vi "Wireless_Serial_Test.vi"() -> ()   [LabVIEW 2010]
uses:
  <vilib>/Instr/_visa.llb/VISA Configure Serial Port (Instr).vi
panel:
  out "Waveform Chart 13":u32(graph)
  out "Waveform Chart 12":u32(graph)
  out "Waveform Chart 11":u32(graph)
  out "Waveform Chart 10":u32(graph)
  out "Waveform Chart 9":u32(graph)
  out "Check Sum":u32(graph)
  out "Waveform Chart 7":u32(graph)
  out "Waveform Chart 6":u32(graph)
  out "Waveform Chart 5":u32(graph)
  out "Waveform Chart 4":u32(graph)
  out "Waveform Chart 3":u32(graph)
  out "Waveform Chart 2":u32(graph)
  out "Waveform Chart":u32(graph)
  in  "byte count":u32=18
  in  "VISA resource name":refnum<visa-resource-name>="COM4"
  in  "stop":bool
  out "Looped Incoming String":string
  out "Active Channels":string
  out "Source Address":string
  out "Byte Length":dbl
  out "RSSI":dbl
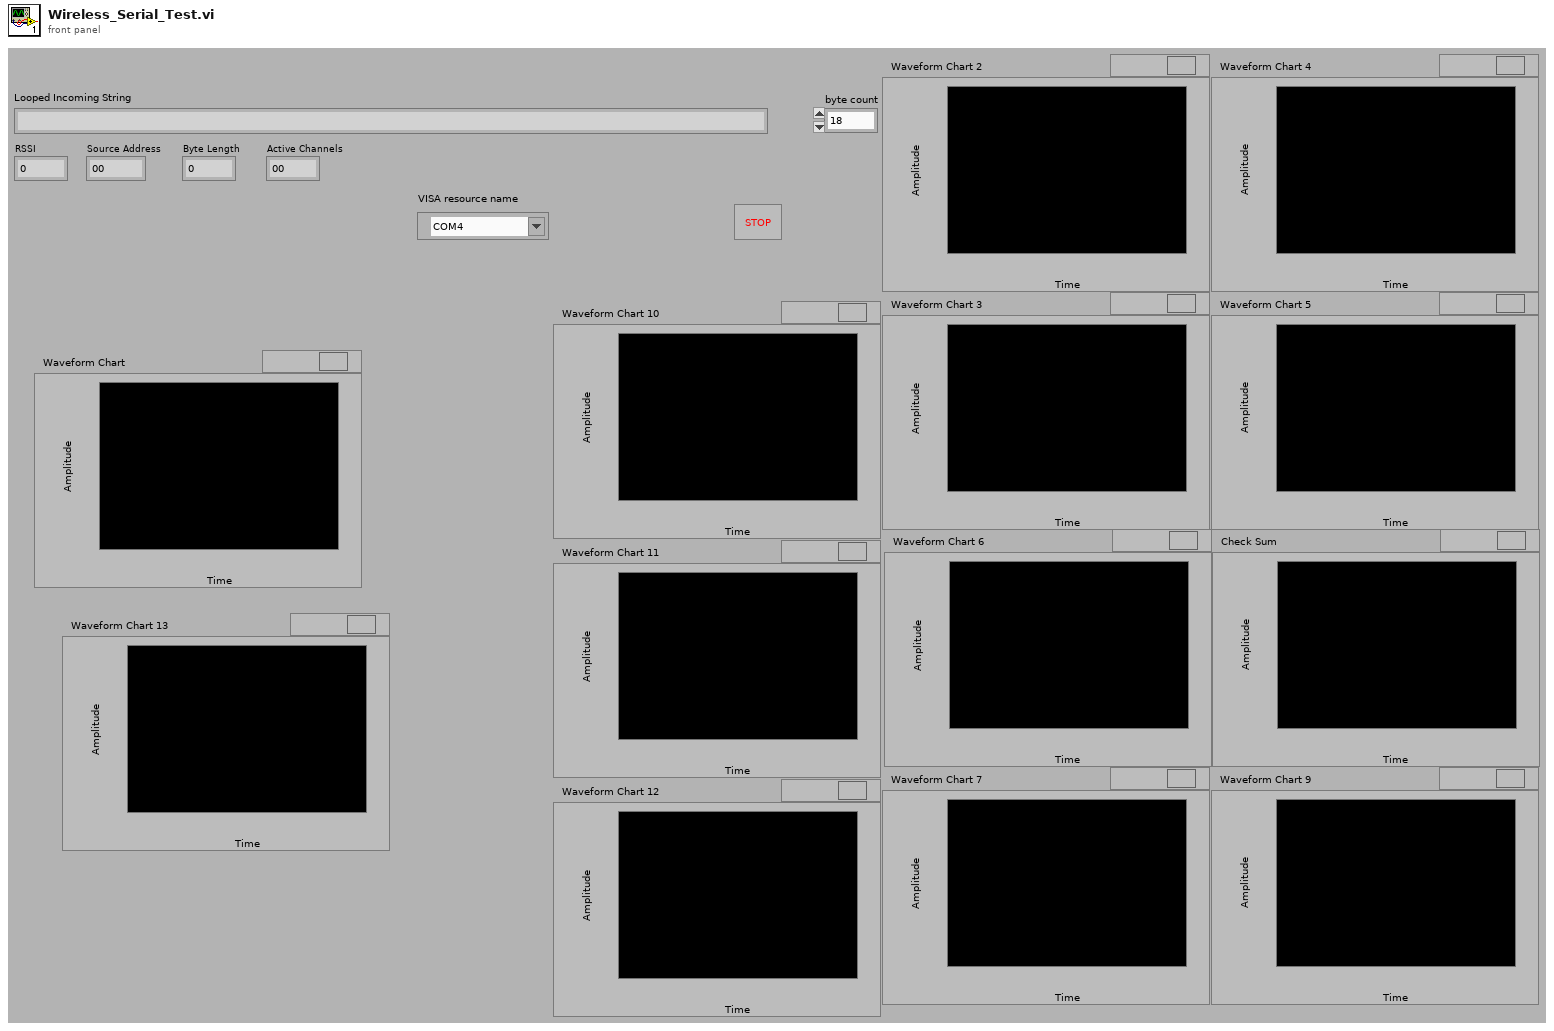
[diagram p1: front panel]
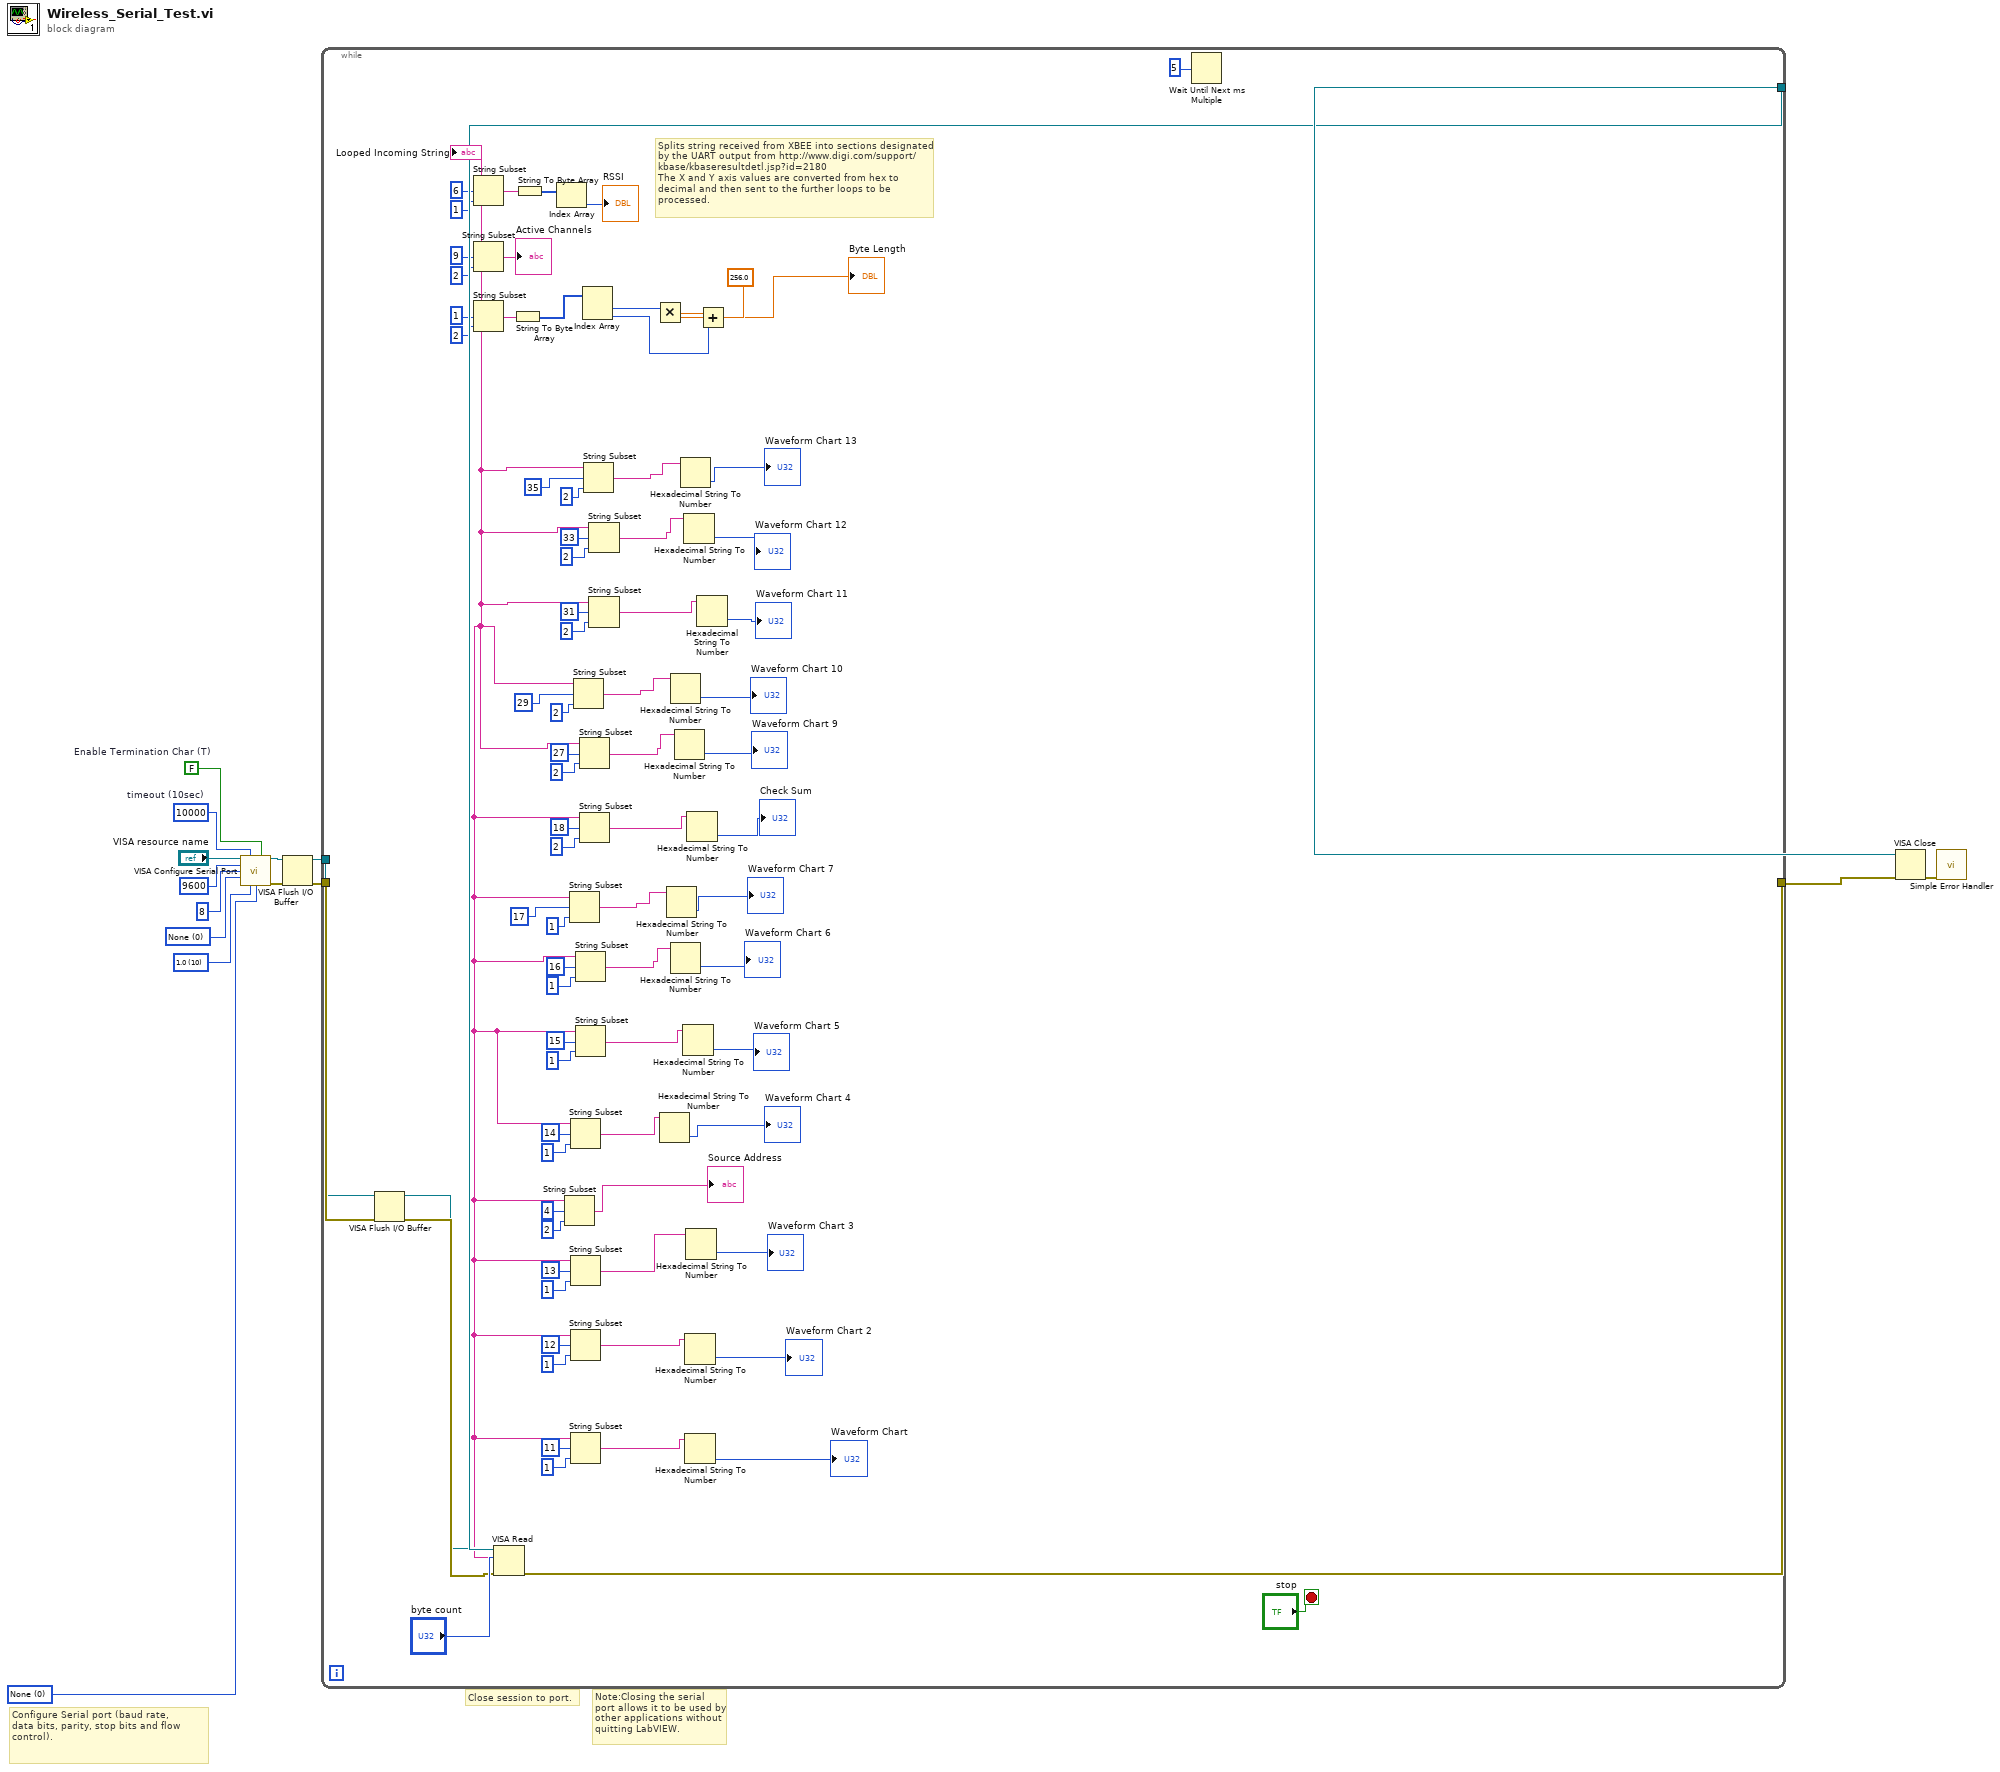
[diagram p0: block diagram]
diagram:
  w4 = u16 0 items=["None"=0, "XON/XOFF"=1, "RTS/CTS"=2, "DTR/DSR"=4] ("flow control")
  w5 = u16 10 items=["1.0"=10, "1.5"=15, "2.0"=20] ("stop bits")
  w8 = u16 0 items=["None", "Odd", "Even", "Mark", "Space"] ("parity")
  w6 = FALSE  # Enable Termination Char (T)
  w7 = u32 10000  # timeout (10sec)
  # "Configure Serial port (baud rate,\ndata bits, parity, stop bits and flow control)."
  # "Note:Closing the serial port allows it to be used by other applications without\nquitting LabVIEW."
  # "Close session to port."
  n1 = call-poly "VISA Configure Serial Port"("VISA resource name"="VISA resource name", "timeout (10sec)"=w7, "Enable Termination\nChar (T)"=w6, "baud rate (9600)"=u32 9600 ("baud rate"), "data bits (8)"=u16 8 ("data bits"), "parity (0:none)"=w8, "stop bits (10: 1 bit)"=w5, "flow control (0:none)"=w4) -> ("VISA resource name out"=w9:refnum<visa-resource-name>, "error out"=w10:errorcluster)  [unwired: 1 in, 5 out]
  n2 = VISA Flush I/O Buffer(VISA resource name=w9, error in (no error)=w10) -> (VISA resource name out=w2:refnum<visa-resource-name>, error out=w1:errorcluster)  [unwired: 1 out]
  n3 = while {
    tunnel: [w97] -> w15
    tunnel: [w96] -> w14
    tunnel: w2 -> [w63]
    tunnel: w1 -> [w64]
    stop <- "stop" stop-if-true
    # "Splits string received from XBEE into sections designated by the UART output from http://www.digi.com/support/kbase/kbaseresultdetl.jsp?id=2180 \nThe X and Y axis values are converted from hex to decimal and then sent to the further loops to be processed."
    n4 = VISA Flush I/O Buffer(VISA resource name=w63, error in (no error)=w64) -> (VISA resource name out=w65:refnum<visa-resource-name>, error out=w66:errorcluster)  [unwired: 1 out]
    n5 = VISA Read(VISA resource name=w65, byte count="byte count", error in (no error)=w66) -> (VISA resource name out=w96:refnum<visa-resource-name>, read buffer=w29:string, error out=w97:errorcluster)  [unwired: 1 out]
    "Looped Incoming String" <- w29
    n6 = String Subset(string=w29, offset (0)=6, length (rest)=1 ("length (rest)")) -> (substring=w68:string)
    n7 = String Subset(string=w29, offset (0)=9, length (rest)=2 ("length (rest)")) -> (substring=→"Active Channels":string)
    n8 = String Subset(string=w29, offset (0)=1, length (rest)=2 ("length (rest)")) -> (substring=w70:string)
    n9 = String To Byte Array(string=w70) -> (unsigned byte array=w72:u8[])
    n10 = String To Byte Array(string=w68) -> (unsigned byte array=w69:u8[])
    n11 = Index Array(array=w69) -> (element=→"RSSI":u8)  [unwired: 1 in]
    n12 = String Subset(string=w29, offset (0)=4, length (rest)=2 ("length (rest)")) -> (substring=→"Source Address":string)
    n13 = String Subset(string=w29, offset (0)=17, length (rest)=1 ("length (rest)")) -> (substring=w54:string)
    n14 = String Subset(string=w29, offset (0)=14, length (rest)=1 ("length (rest)")) -> (substring=w51:string)
    n15 = String Subset(string=w29, offset (0)=13, length (rest)=1 ("length (rest)")) -> (substring=w50:string)
    n16 = String Subset(string=w29, offset (0)=12, length (rest)=1 ("length (rest)")) -> (substring=w49:string)
    n17 = String Subset(string=w29, offset (0)=11, length (rest)=1 ("length (rest)")) -> (substring=w48:string)
    n18 = String Subset(string=w29, offset (0)=29, length (rest)=2 ("length (rest)")) -> (substring=w41:string)
    n19 = String Subset(string=w29, offset (0)=16, length (rest)=1 ("length (rest)")) -> (substring=w53:string)
    n20 = String Subset(string=w29, offset (0)=15, length (rest)=1 ("length (rest)")) -> (substring=w52:string)
    n21 = String Subset(string=w29, offset (0)=27, length (rest)=2 ("length (rest)")) -> (substring=w40:string)
    n22 = String Subset(string=w29, offset (0)=18, length (rest)=2 ("length (rest)")) -> (substring=w39:string)
    n23 = Index Array(array=w72) -> (element #1=w75:u8, element #2=w73:u8)  [unwired: 2 in]
    n24 = String Subset(string=w29, offset (0)=35, length (rest)=2 ("length (rest)")) -> (substring=w32:string)
    n25 = String Subset(string=w29, offset (0)=33, length (rest)=2 ("length (rest)")) -> (substring=w31:string)
    n26 = String Subset(string=w29, offset (0)=31, length (rest)=2 ("length (rest)")) -> (substring=w30:string)
    n27 = Multiply(x=w75, y=256.0) -> (x*y=w74:dbl)
    n28 = Hexadecimal String To Number(string=w51) -> (number=→"Waveform Chart 4":u32)  [unwired: 3 out]
    n29 = Hexadecimal String To Number(string=w54) -> (number=→"Waveform Chart 7":u32)  [unwired: 3 out]
    n30 = Hexadecimal String To Number(string=w41) -> (number=→"Waveform Chart 10":u32)  [unwired: 3 out]
    n31 = Hexadecimal String To Number(string=w53) -> (number=→"Waveform Chart 6":u32)  [unwired: 3 out]
    n32 = Hexadecimal String To Number(string=w40) -> (number=→"Waveform Chart 9":u32)  [unwired: 3 out]
    n33 = Hexadecimal String To Number(string=w32) -> (number=→"Waveform Chart 13":u32)  [unwired: 3 out]
    n34 = Hexadecimal String To Number(string=w52) -> (number=→"Waveform Chart 5":u32)  [unwired: 3 out]
    n35 = Hexadecimal String To Number(string=w31) -> (number=→"Waveform Chart 12":u32)  [unwired: 3 out]
    n36 = Hexadecimal String To Number(string=w49) -> (number=→"Waveform Chart 2":u32)  [unwired: 3 out]
    n37 = Hexadecimal String To Number(string=w48) -> (number=→"Waveform Chart":u32)  [unwired: 3 out]
    n38 = Hexadecimal String To Number(string=w50) -> (number=→"Waveform Chart 3":u32)  [unwired: 3 out]
    n39 = Hexadecimal String To Number(string=w39) -> (number=→"Check Sum":u32)  [unwired: 3 out]
    n40 = Hexadecimal String To Number(string=w30) -> (number=→"Waveform Chart 11":u32)  [unwired: 3 out]
    n41 = Add(x=w74, y=w73) -> (x+y=→"Byte Length":dbl)
    n42 = Wait Until Next ms Multiple(millisecond multiple=u32 5 ("milliseconds to wait")) -> ()  [unwired: 1 out]
  }
  n43 = VISA Close(VISA resource name=w14, error in (no error)=w15) -> (error out=w13:errorcluster)
  n44 = call <vilib>:"Simple Error Handler.vi"("error in (no error)"=w13) -> ()  [unwired: 1 in, 8 out]
